vi "Create Events.vi"(8 "error in (no error)":errorcluster, 11 "RPI.SenseHat.Actor in":refnum<class "RPI.SenseHat.Actor.lvclass">) -> (0 "error out":errorcluster, 3 "RPI.SenseHat.Actor out":refnum<class "RPI.SenseHat.Actor.lvclass">)   [LabVIEW 2020, in "RPI.SenseHat.Actor.lvlib" / "RPI.SenseHat.Actor.lvclass"]
uses:
  RPI.SenseHat.Actor.lvclass
  RPI.SenseHat.Joystick/TypeDefs/Joystick.ctl
  Protected Events.ctl
  Public Events.ctl
  RPI.SenseHat.Actor.lvclass/RPI.SenseHat.Actor.ctl
  RPI.SenseHat.Joystick/RPI.SenseHat.Joystick.lvlib
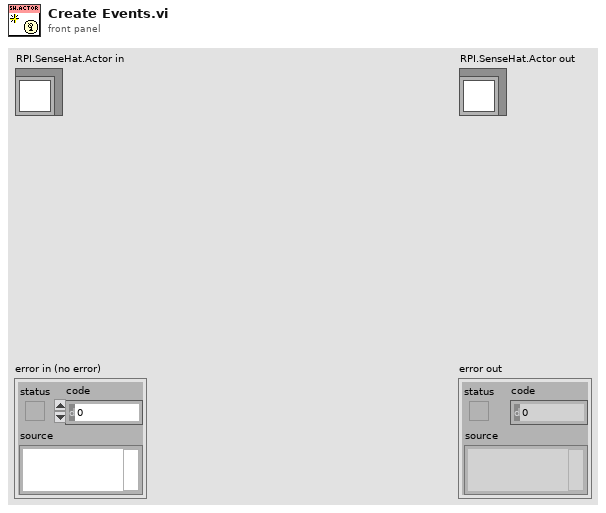
[diagram p1: front panel]
types:
  T1 = typedef "RPI.SenseHat.Actor.lvlib/RPI.SenseHat.Actor.lvclass/Public Events.ctl" = cluster{"Joystick Update":refnum<user-event>}
  T2 = typedef "RPI.SenseHat.Actor.lvlib/RPI.SenseHat.Actor.lvclass/Protected Events.ctl" = cluster{"StopActor":refnum<user-event>}
  T3 = typedef "RPI.SenseHat.Joystick.lvlib/Joystick.ctl" = cluster{"Enter":bool, "Down":bool, "Up":bool, "Right":bool, "Left":bool}
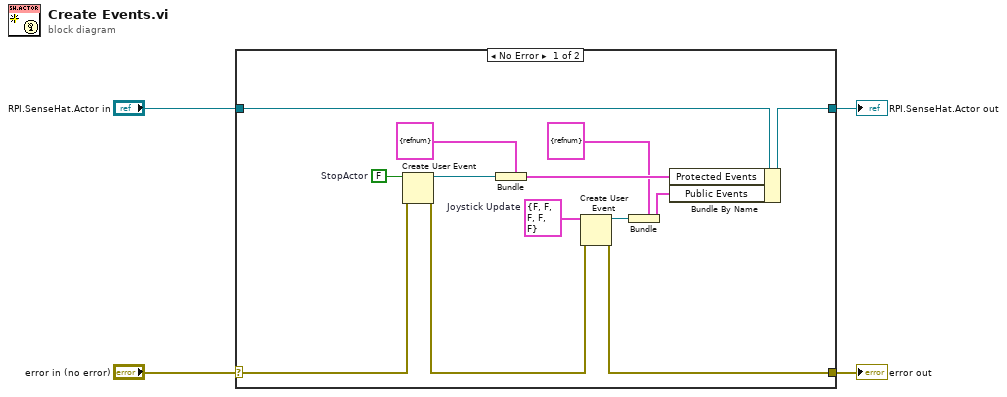
[diagram p0: block diagram]
diagram:
  n1 = case shown="No Error" "error in (no error)" {
    selector: "error in (no error)" -> [w12 w19]
    tunnel: [w7 w19] -> w3
    tunnel: [w16 w18] -> w1
    tunnel: "RPI.SenseHat.Actor in" -> [w17 w18]
    frame No Error {
      w9 = T3 {"Enter"=FALSE, "Down"=FALSE, "Up"=FALSE, "Right"=FALSE, "Left"=FALSE}  # Joystick Update
      w15 = FALSE  # StopActor
      n2 = Create User Event(user event datatype=w15, error in=w12) -> (user event=w14:refnum<user-event>, error out=w8:errorcluster)
      n3 = Bundle(cluster=T2 {"StopActor"=refnum} ("Protected Events"), "StopActor"=w14) -> (w13:T2)
      n4 = Create User Event(user event datatype=w9, error in=w8) -> (user event=w11:refnum<user-event>, error out=w7:errorcluster)
      n5 = Bundle(cluster=T1 {"Joystick Update"=refnum} ("Public Events"), "Joystick Update"=w11) -> (w10:T1)
      n6 = Bundle By Name(cluster=w17, "Protected Events"=w13, "Public Events"=w10) -> (w16:refnum<class "RPI.SenseHat.Actor.lvclass">)
    }
    frame Error {
    }
  }
  "error out" <- w3
  "RPI.SenseHat.Actor out" <- w1
